vi "Poly Roots for PFE (CDB).vi"(11 "P(x)":cdb[](array[numeric]) format="%#.6g") -> (3 "Roots":cdb[](array[numeric]))   [LabVIEW 2017, in "NI_AALPro.lvlib"]
uses:
  NI_AALPro.lvlib
  Eigenvalue and Vectors Output Option.ctl
  RMS (CDB).vi
  RMS (DBL).vi
  Create Polynomial From Roots (CDB).vi
  Polynomial Roots (DBL).vi
  Real Eigenvalues and Vectors.vi
  Create Special Real Matrix.vi
  Polynomial Roots (CDB).vi
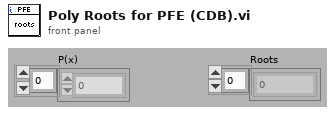
[diagram p1: front panel]
types:
  T1 = enum32{"Identity", "Diagonal", "Toepliz", "Vandermonde", "Companion"}
  T2 = typedef "NI_AALPro.lvlib/Eigenvalue and Vectors Output Option.ctl" = i32
  T3 = typedef "NI_Matrix.lvlib/RealMatrix.ctl" = dbl[][]
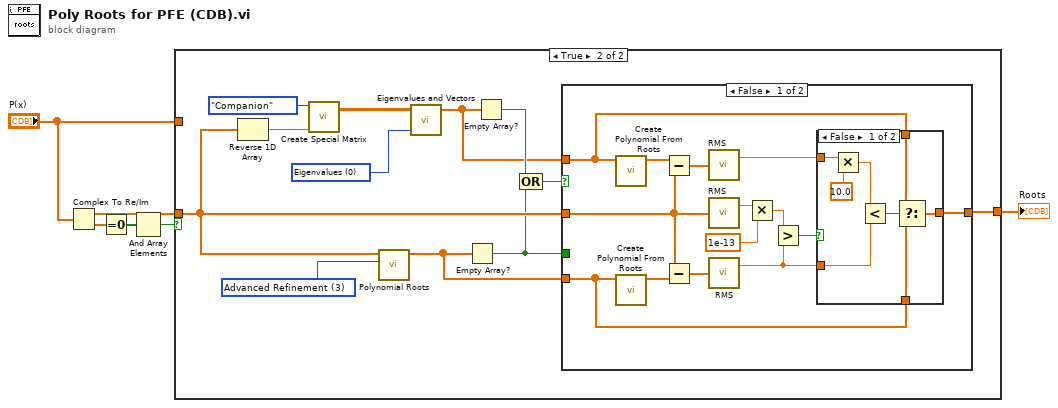
[diagram p0: block diagram]
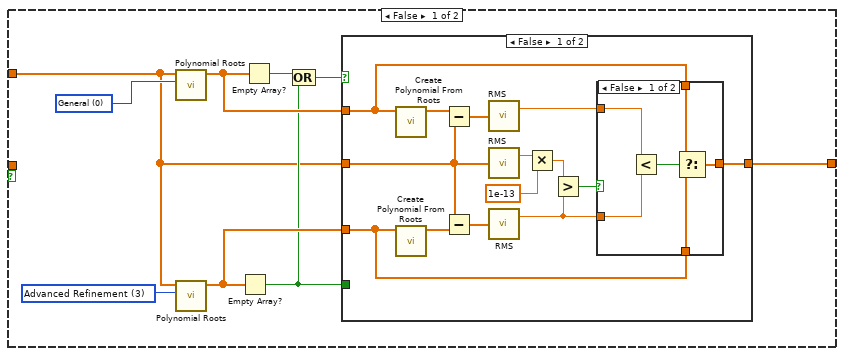
[diagram p2: hidden frame]
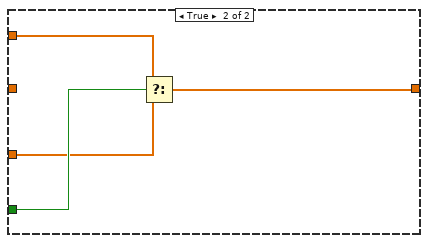
[diagram p4: hidden frame]
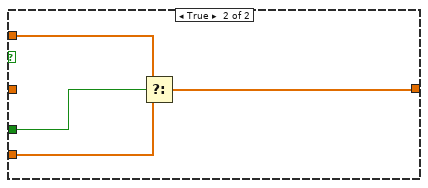
[diagram p6: hidden frame]
diagram:
  n1 = Complex To Re/Im(x + iy="P(x)") -> (x=w1:dbl[], y=w4:dbl[])
  n2 = Equal To 0?(x=w4) -> (x = 0?=w3:bool[])
  n3 = And Array Elements(Boolean array=w3) -> (logical AND=w2:bool)
  n4 = case shown="True" w2 {
    tunnel: [w8 w42] -> w6
    tunnel: "P(x)" -> [w7 _]
    tunnel: w1 -> [_ w43]
    frame False {
      w14 = u16 3 items=["General"=0, "Advanced Refinement"=3] ("option")
      w15 = u16 0 items=["General"=0, "Advanced Refinement"=3] ("option")
      n5 = call-poly "Polynomial Roots.vi"("option"=w15, "P(x)"=w7) -> ("Roots"=w13:cdb[])  [unwired: 8 in, 1 out]
      n6 = call-poly "Polynomial Roots.vi"("option"=w14, "P(x)"=w7) -> ("Roots"=w12:cdb[])  [unwired: 8 in, 1 out]
      n7 = Empty Array?(array=w12) -> (empty?=w9:bool)
      n8 = Empty Array?(array=w13) -> (empty?=w10:bool)
      n9 = Compound Arithmetic op=OR(w10, w9) -> (w11:bool)
      n10 = case shown="False" w11 {
        tunnel: w13 -> [w26 w39]
        tunnel: w12 -> [w25 w38]
        tunnel: w7 -> [w23 _]
        tunnel: w9 -> [_ w40]
        tunnel: [w24 w37] -> w8
        frame False {
          n11 = call-poly "Create Polynomial From Roots.vi"("Roots"=w26) -> ("P(x)"=w28:cdb[])  [unwired: 9 in, 1 out]
          n12 = call-poly "Create Polynomial From Roots.vi"("Roots"=w25) -> ("P(x)"=w29:cdb[])  [unwired: 9 in, 1 out]
          n13 = Subtract(x=w28, y=w23) -> (x-y=w22:cdb[])
          n14 = Subtract(x=w23, y=w29) -> (x-y=w21:cdb[])
          n15 = call-poly "RMS.vi"("X"=w22) -> ("rms value"=w27:dbl)  [unwired: 1 out]
          n16 = call-poly "RMS.vi"("X"=w23) -> ("rms value"=w20:dbl)  [unwired: 1 out]
          n17 = call-poly "RMS.vi"("X"=w21) -> ("rms value"=w17:dbl)  [unwired: 1 out]
          n18 = Multiply(x=w20, y=1e-13) -> (x*y=w18:dbl)
          n19 = Greater?(x=w18, y=w17) -> (0:w16:bool)
          n20 = case shown="False" w16 {
            tunnel: w27 -> [w35 _]
            tunnel: w26 -> [w33 _]
            tunnel: w25 -> [w32 w36]
            tunnel: [w31 w36] -> w24
            tunnel: w17 -> [w30 _]
            frame False {
              n21 = Less?(x=w35, y=w30) -> (x < y?=w34:bool)
              n22 = Select(t=w33, s=w34, f=w32) -> (s? t:f=w31:cdb[])
            }
            frame True {
            }
          }
        }
        frame True {
          n23 = Select(t=w39, s=w40, f=w38) -> (s? t:f=w37:cdb[])
        }
      }
    }
    frame True {
      w48 = T2 0 items=["Eigenvalues", "Eigenvalues & Vectors"] ("output option")
      w52 = u16 3 items=["General", "Simple Classification", "Refinement", "Advanced Refinement"] ("option")
      n24 = Reverse 1D Array(array=w43) -> (reversed array=w51:dbl[])
      n25 = call-poly "Create Special Matrix.vi"("matrix type"=T1."Companion", "Input Vector1"=w51) -> ("Special Matrix"=w49:T3)  [unwired: 3 in, 1 out]
      n26 = call-poly "Polynomial Roots.vi"("option"=w52, "P(x)"=w43) -> ("Roots"=w44:cdb[])  [unwired: 8 in, 1 out]
      n27 = call-poly "Eigenvalues and Vectors.vi"("output option"=w48, "Input Matrix"=w49) -> ("Eigenvalues"=w45:cdb[])  [unwired: 1 in, 2 out]
      n28 = Empty Array?(array=w44) -> (empty?=w41:bool)
      n29 = Empty Array?(array=w45) -> (empty?=w47:bool)
      n30 = Compound Arithmetic op=OR(w47, w41) -> (w46:bool)
      n31 = case shown="False" w46 {
        tunnel: w45 -> [w63 w79]
        tunnel: w44 -> [w62 w78]
        tunnel: w43 -> [w60 _]
        tunnel: [w61 w77] -> w42
        tunnel: w41 -> [_ w76]
        frame False {
          n32 = call-poly "Create Polynomial From Roots.vi"("Roots"=w63) -> ("P(x)"=w65:cdb[])  [unwired: 9 in, 1 out]
          n33 = call-poly "Create Polynomial From Roots.vi"("Roots"=w62) -> ("P(x)"=w66:cdb[])  [unwired: 9 in, 1 out]
          n34 = Subtract(x=w65, y=w60) -> (x-y=w59:cdb[])
          n35 = Subtract(x=w60, y=w66) -> (x-y=w58:cdb[])
          n36 = call-poly "RMS.vi"("X"=w59) -> ("rms value"=w64:dbl)  [unwired: 1 out]
          n37 = call-poly "RMS.vi"("X"=w60) -> ("rms value"=w57:dbl)  [unwired: 1 out]
          n38 = call-poly "RMS.vi"("X"=w58) -> ("rms value"=w54:dbl)  [unwired: 1 out]
          n39 = Multiply(x=w57, y=1e-13) -> (x*y=w55:dbl)
          n40 = Greater?(x=w55, y=w54) -> (0:w53:bool)
          n41 = case shown="False" w53 {
            tunnel: w64 -> [w69 _]
            tunnel: w63 -> [w73 _]
            tunnel: w62 -> [w72 w75]
            tunnel: [w71 w75] -> w61
            tunnel: w54 -> [w70 _]
            frame False {
              n42 = Multiply(x=w69, y=10.0) -> (x*y=w68:dbl)
              n43 = Less?(x=w68, y=w70) -> (x < y?=w74:bool)
              n44 = Select(t=w73, s=w74, f=w72) -> (s? t:f=w71:cdb[])
            }
            frame True {
            }
          }
        }
        frame True {
          n45 = Select(t=w79, s=w76, f=w78) -> (s? t:f=w77:cdb[])
        }
      }
    }
  }
  "Roots" <- w6
